vi "Spartan HTTP Load Configuration Files.vi"(4 "error in":errorcluster, 7 "lvhttp.cfg":path=path "") -> (0 "error out":errorcluster, 3 "Config Load Message":string)   [LabVIEW 2011]
uses:
  server lib/Spartan Version.vi
  ITK EXT/http/config.llb/HTTP SRM.vi
  ITK EXT/http/http0.llb/HTTP LVHTTP Global.vi
  ITK EXT/http/http0.llb/HTTP Server Globals.glb
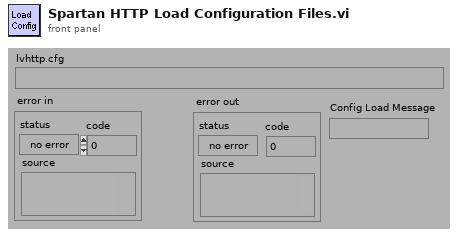
[diagram p1: front panel]
types:
  T1 = typedef "Keyed Array.ctl" = cluster{"keys":string[], "values":string[]}
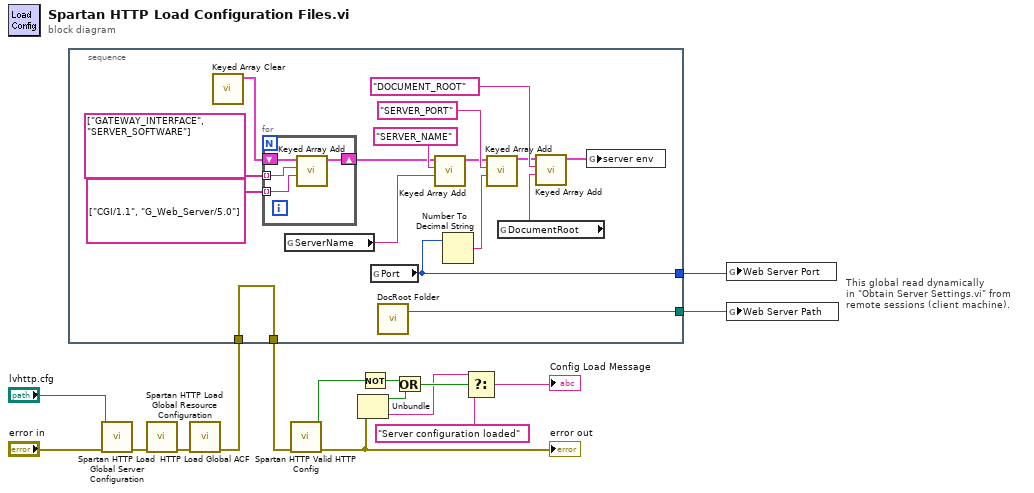
[diagram p0: block diagram]
diagram:
  # "This global read dynamically\nin \"Obtain Server Settings.vi\" from\nremote sessions (client machine)."
  n1 = call "Spartan HTTP Load Global Server Configuration.vi"("error in (no error)"="error in", "lvhttp.conf"="lvhttp.cfg") -> ("error out"=w16:errorcluster)  [unwired: 9 out]
  n2 = call "Spartan HTTP Load Global Resource Configuration.vi"("error in (no error)"=w16) -> ("error out"=w15:errorcluster)  [unwired: 10 out]
  n3 = call "HTTP Load Global ACF.vi"("error in (no error)"=w15) -> ("error out"=w12:errorcluster)  [unwired: 6 out]
  n4 = stacked-sequence {
    tunnel: w12 -> [w20]
    tunnel: [w20] -> w11
    tunnel: [w18] -> w2
    tunnel: [w17] -> w1
    frame #0 {
      n5 = call "Keyed Array Clear.vi"() -> ("array out"=w22:T1)  [unwired: 1 in, 6 out]
      n6 = for {
        shift-right: [w34] -> w27
        shift-left: w22 -> [w35]
        tunnel: string[] ["GATEWAY_INTERFACE", "SERVER_SOFTWARE"] -> [w36] mode=indexing
        tunnel: string[] ["CGI/1.1", "G_Web_Server/5.0"] -> [w33] mode=indexing
        n7 = call "Keyed Array Add.vi"("value"=w33, "key"=w36, "array in"=w35) -> ("array out"=w34:T1)  [unwired: 1 in, 3 out]
      }
      n8 = global read "HTTP LVHTTP Global.vi" "ServerName"() -> (w23:string)
      n9 = global read "HTTP LVHTTP Global.vi" "Port"() -> (w18:u16)
      n10 = call "DocRoot Folder.vi"() -> ("DocumentRoot Folder"=w17:path)  [unwired: 3 in]
      n11 = call "Keyed Array Add.vi"("value"=w23, "key"="SERVER_NAME", "array in"=w27) -> ("array out"=w24:T1)  [unwired: 1 in, 3 out]
      n12 = Number To Decimal String(number=w18) -> (decimal integer string=w21:string)  [unwired: 1 out]
      n13 = call "Keyed Array Add.vi"("value"=w21, "key"="SERVER_PORT", "array in"=w24) -> ("array out"=w25:T1)  [unwired: 1 in, 3 out]
      n14 = global read "HTTP SRM.vi" "DocumentRoot"() -> (w19:string)
      n15 = call "Keyed Array Add.vi"("value"=w19, "key"="DOCUMENT_ROOT", "array in"=w25) -> ("array out"=w26:T1)  [unwired: 1 in, 3 out]
      n16 = global write "HTTP Server Globals.glb" "server env"(w26) -> ()
    }
  }
  n17 = call "Spartan HTTP Valid HTTP Config.vi"("error in (no error)"=w11) -> ("error out"=w10:errorcluster, "valid"=w8:bool)  [unwired: 9 out]
  "error out" <- w10
  n18 = Unbundle(w10) -> ("status"=w9:bool, "source"=w5:string)  [unwired: 1 out]
  n19 = Not(x=w8) -> (.not. x?=w7:bool)
  n20 = Or(x=w7, y=w9) -> (x .or. y?=w6:bool)
  n21 = Select(t=w5, s=w6, f="Server configuration loaded" ("source")) -> (s? t:f=→"Config Load Message":string)
  n22 = global write "Spartan Version.vi" "Web Server Port"(w2) -> ()
  n23 = global write "Spartan Version.vi" "Web Server Path"(w1) -> ()
